vi "laserInit.vi"(8 "error in (no error)":errorcluster, 10 "LaserPropIn":T2, 11 "LaserIn":T1) -> (0 "error out":errorcluster, 2 "LaserOut":T1, 3 "LaserPropOut":T2)   [LabVIEW 2021]
uses:
  Users/Fred/Desktop/CoboltLaserDrivers_Public_LV2021/CoboltLaserDrivers_Public/CoboltLaser_Controls/ExpectedResponseType.ctl
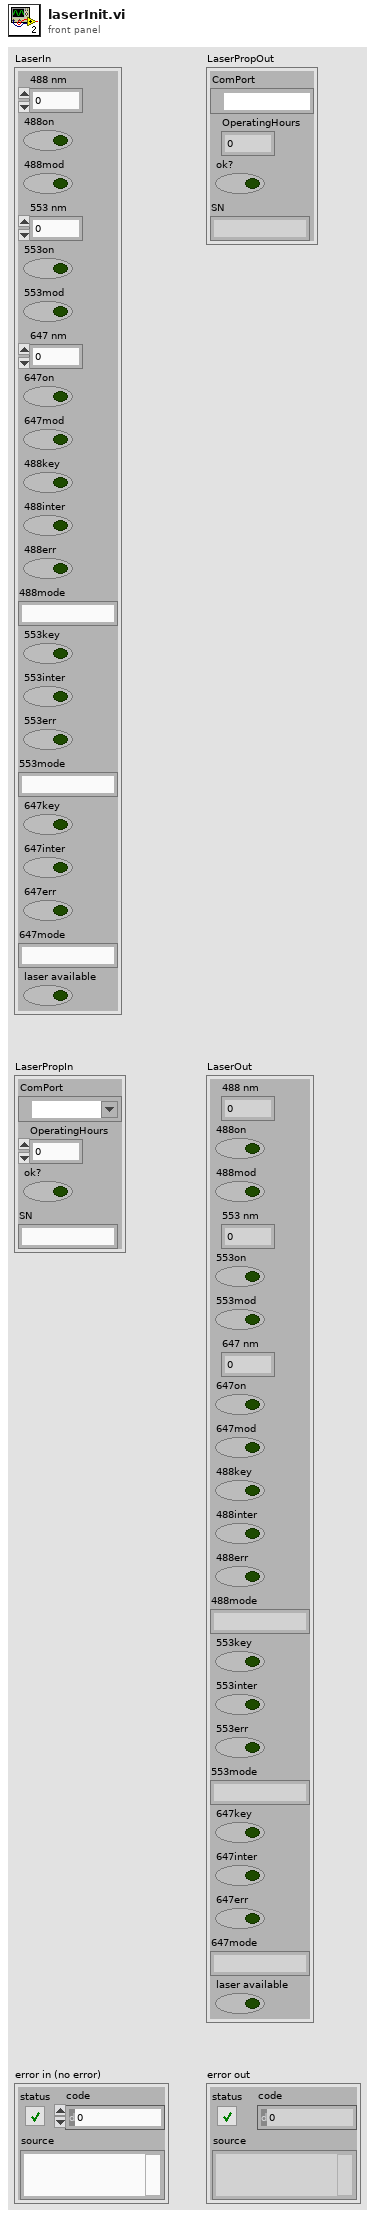
[diagram p1: front panel]
types:
  T1 = cluster{"488 nm":dbl, "488on":bool, "488mod":bool, "553 nm":dbl, "553on":bool, "553mod":bool, "647 nm":dbl, "647on":bool, "647mod":bool, "488key":bool, "488inter":bool, "488err":bool, "488mode":string, "553key":bool, "553inter":bool, "553err":bool, "553mode":string, "647key":bool, "647inter":bool, "647err":bool, "647mode":string, "laser available":bool}
  T2 = cluster{"ComPort":refnum<visa-resource-name>, "OperatingHours":dbl, "ok?":bool, "SN":string}
  T3 = typedef "ExpectedResponseType.ctl" = enum16{"Any", "Digits Only", "Non-Digits Only"}
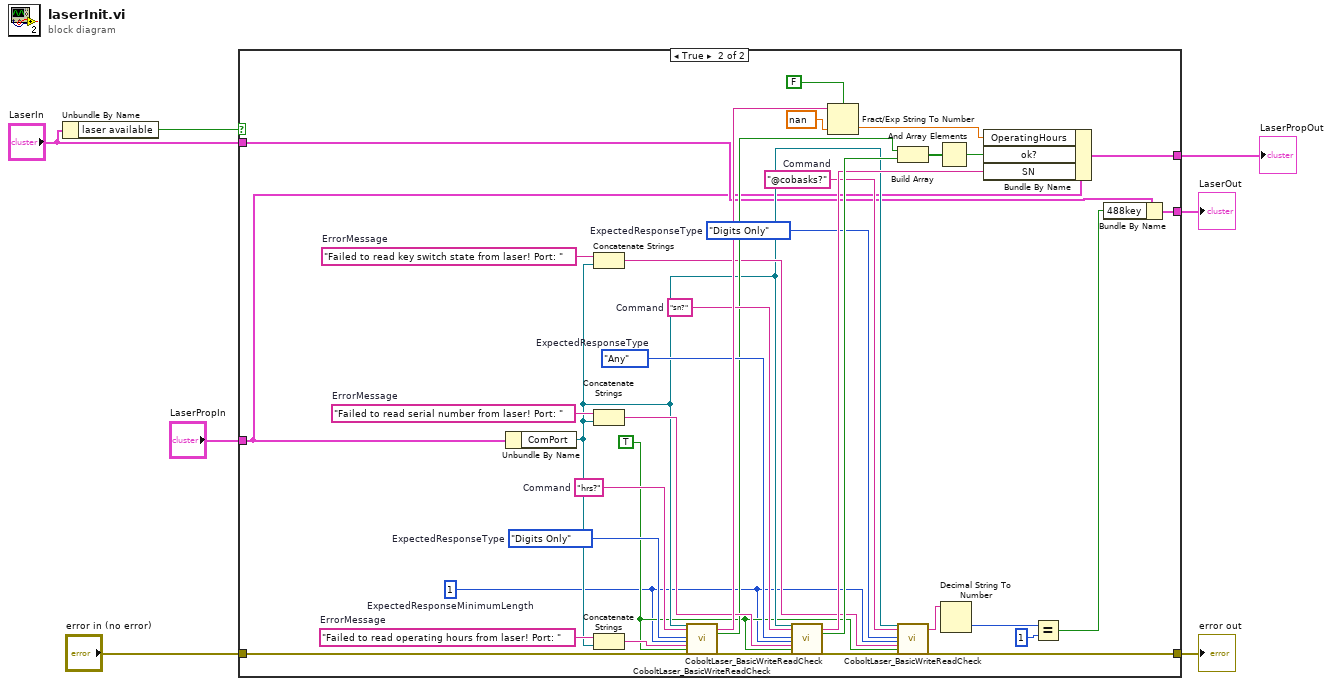
[diagram p0: block diagram]
diagram:
  n1 = Unbundle By Name("LaserIn") -> ("laser available"=w3:bool)
  n2 = case shown="True" w3 {
    tunnel: "error in (no error)" -> [w10 w39]
    tunnel: [w10 w11] -> w2
    tunnel: "LaserIn" -> [w9 w17]
    tunnel: [w9 w15] -> w5
    tunnel: [w8 w14] -> w6
    tunnel: "LaserPropIn" -> [w8 w13]
    frame False {
    }
    frame True {
      w26 = enum16{"Any", "Digits Only", "Non-Digits Only"}."Digits Only"  # ExpectedResponseType
      w25 = "Failed to read key switch state from laser! Port: "  # ErrorMessage
      w27 = "@cobasks?"  # Command
      w34 = ExpectedResponseType."Any"  # ExpectedResponseType
      w36 = "Failed to read serial number from laser! Port: "  # ErrorMessage
      w37 = "sn?"  # Command
      w19 = TRUE ("GenerateError")
      w42 = ExpectedResponseType."Digits Only"  # ExpectedResponseType
      w18 = 1  # ExpectedResponseMinimumLength
      w45 = "Failed to read operating hours from laser! Port: "  # ErrorMessage
      w46 = "hrs?"  # Command
      n3 = Unbundle By Name(w13) -> ("ComPort"=w20:refnum<visa-resource-name>)
      n4 = Concatenate Strings(w25, w20) -> (w24:string)
      n5 = Concatenate Strings(w36, w20) -> (w35:string)
      n6 = Concatenate Strings(w45, w20) -> (w44:string)
      n7 = call "CoboltLaser_BasicWriteReadCheck.vi"("ComPort"=w20, "Command"=w46, "ExpectedResponseType"=w42, "ExpectedResponseMinimumLength"=w18, "ErrorMessage"=w44, "GenerateError"=w19, "error in (no error)"=w39) -> ("Response"=w40:string, "ResponseOK"=w31:bool, "error out"=w33:errorcluster)  [unwired: 17 in, 1 out]
      n8 = call "CoboltLaser_BasicWriteReadCheck.vi"("ComPort"=w20, "Command"=w37, "ExpectedResponseType"=w34, "ExpectedResponseMinimumLength"=w18, "ErrorMessage"=w35, "GenerateError"=w19, "error in (no error)"=w33) -> ("Response"=w29:string, "ResponseOK"=w30:bool, "error out"=w12:errorcluster)  [unwired: 17 in, 1 out]
      n9 = Fract/Exp String To Number(use system decimal point (T)=FALSE, string=w40, default (0 dbl)=nan ("default (0 DBL)")) -> (number=w38:dbl)  [unwired: 1 in, 1 out]
      n10 = Build Array(w31, w30) -> (w28:bool[])
      n11 = call "CoboltLaser_BasicWriteReadCheck.vi"("ComPort"=w20, "Command"=w27, "ExpectedResponseType"=w26, "ExpectedResponseMinimumLength"=w18, "ErrorMessage"=w24, "GenerateError"=w19, "error in (no error)"=w12) -> ("Response"=w23:string, "error out"=w11:errorcluster)  [unwired: 17 in, 2 out]
      n12 = And Array Elements(Boolean array=w28) -> (logical AND=w32:bool)
      n13 = Decimal String To Number(string=w23) -> (number=w22:i32)  [unwired: 2 in, 1 out]
      n14 = Bundle By Name(cluster=w13, "OperatingHours"=w38, "ok?"=w32, "SN"=w29) -> (w14:T2)
      n15 = Equal?(x=w22, y=1) -> (x = y?=w16:bool)
      n16 = Bundle By Name(cluster=w17, "488key"=w16) -> (w15:T1)
    }
  }
  "LaserPropOut" <- w6
  "LaserOut" <- w5
  "error out" <- w2
